vi "Liczniki.vi"() -> ()   [LabVIEW 2017, in "GUI.lvlib"]
uses:
  Libraries/GUI/GUI.lvlib
  <vilib>/Utility/config.llb/NI_LVConfig.lvlib
panel:
  out "Slave 2":T1
  out "Slave 6":T2
  out "Slave 4":T3
  out "Slave 3":T4
  out "Slave 5":T5
  in  "P_Sx":T6
  in  "stop":bool
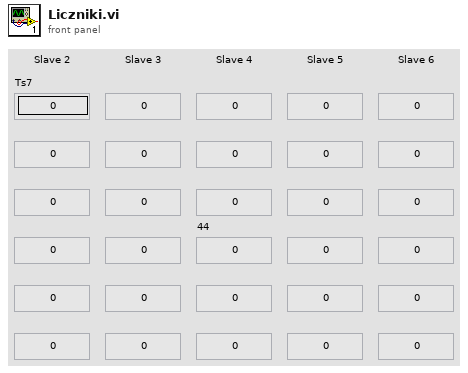
[diagram p1: front panel]
types:
  T1 = cluster{"Zmienna 11":dbl, "Zmienna 12":dbl, "Zmienna 13":dbl, "Zmienna 14":dbl, "Zmienna 15":dbl, "Zmienna 16":dbl}
  T2 = cluster{"Zmienna 51":dbl, "Zmienna 52":dbl, "Zmienna 53":dbl, "Zmienna 54":dbl, "Zmienna 55":dbl, "Zmienna 56":dbl}
  T3 = cluster{"Zmienna 31":dbl, "Zmienna 32":dbl, "Zmienna 33":dbl, "Zmienna 34":dbl, "Zmienna 35":dbl, "Zmienna 36":dbl}
  T4 = cluster{"Zmienna 21":dbl, "Zmienna 22":dbl, "Zmienna 23":dbl, "Zmienna 24":dbl, "Zmienna 25":dbl, "Zmienna 26":dbl}
  T5 = cluster{"Zmienna 41":dbl, "Zmienna 42":dbl, "Zmienna 43":dbl, "Zmienna 44":dbl, "Zmienna 45":dbl, "Zmienna 46":dbl}
  T6 = cluster{"Stan 1":dbl, "Stan 2":dbl, "Stan 3":dbl, "Stan 4":dbl, "Stan 5":dbl, "Stan 6":dbl}
  T7 = cluster{"Controls[]":refnum<vi>[], "Controls[]":refnum<vi>[], "Controls[]":refnum<vi>[], "Controls[]":refnum<vi>[], "Controls[]":refnum<vi>[], "Controls[]":refnum<vi>[]}
  T8 = typedef "NI_LVConfig.lvlib/Config Data RefNum.ctl" = refnum<k1>
  T9 = cluster{"[0]":cluster{"Stan 1":dbl, "Stan 2":dbl, "Stan 3":dbl, "Stan 4":dbl, "Stan 5":dbl, "Stan 6":dbl}, "[1]":cluster{"Stan 1":dbl, "Stan 2":dbl, "Stan 3":dbl, "Stan 4":dbl, "Stan 5":dbl, "Stan 6":dbl}, "[2]":cluster{"Stan 1":dbl, "Stan 2":dbl, "Stan 3":dbl, "Stan 4":dbl, "Stan 5":dbl, "Stan 6":dbl}, "[3]":cluster{"Stan 1":dbl, "Stan 2":dbl, "Stan 3":dbl, "Stan 4":dbl, "Stan 5":dbl, "Stan 6":dbl}, "[4]":cluster{"Stan 1":dbl, "Stan 2":dbl, "Stan 3":dbl, "Stan 4":dbl, "Stan 5":dbl, "Stan 6":dbl}}
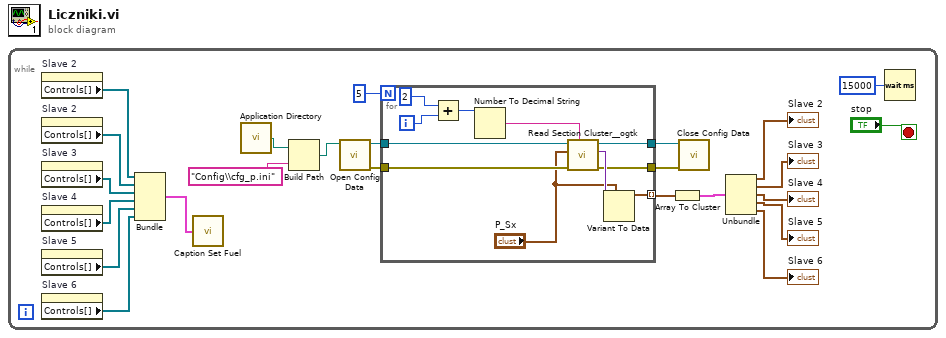
[diagram p0: block diagram]
diagram:
  n1 = while {
    stop <- "stop" stop-if-true
    n2 = property on="Slave 2" class="Clust (strict)"() -> ("Controls[]"=w1:refnum<vi>[])  [unwired: 2 in, 2 out]
    n3 = property on="Slave 2" class="Clust (strict)"() -> ("Controls[]"=w2:refnum<vi>[])  [unwired: 2 in, 2 out]
    n4 = property on="Slave 3" class="Clust (strict)"() -> ("Controls[]"=w3:refnum<vi>[])  [unwired: 2 in, 2 out]
    n5 = property on="Slave 4" class="Clust (strict)"() -> ("Controls[]"=w6:refnum<vi>[])  [unwired: 2 in, 2 out]
    n6 = property on="Slave 5" class="Clust (strict)"() -> ("Controls[]"=w5:refnum<vi>[])  [unwired: 2 in, 2 out]
    n7 = property on="Slave 6" class="Clust (strict)"() -> ("Controls[]"=w4:refnum<vi>[])  [unwired: 2 in, 2 out]
    n8 = Bundle("Controls[]"=w1, "Controls[]"=w2, "Controls[]"=w3, "Controls[]"=w6, "Controls[]"=w5, "Controls[]"=w4) -> (w7:T7)  [unwired: 1 in]
    n9 = call "Caption Set Fuel.vi"("Reference Cluster"=w7) -> ()
    n10 = call <vilib>:"Application Directory.vi"() -> ("Application Directory"=w22:path)
    n11 = Build Path(base path=w22, name or relative path="Config\\cfg_p.ini") -> (appended path=w20:path)
    n12 = call <vilib>:"Open Config Data.vi"("configuration file path"=w20) -> ("error out"=w18:errorcluster, "refnum"=w19:T8)  [unwired: 8 in, 1 out]
    n13 = for {
      N: 5 -> [_]
      tunnel: w19 -> [w34]
      tunnel: w18 -> [w33]
      tunnel: [w27] -> w16 mode=indexing
      tunnel: [w26] -> w9
      tunnel: [w25] -> w8
      i -> [w32]
      n14 = Add(x=2, y=w32) -> (x+y=w29:i32)
      n15 = Number To Decimal String(number=w29) -> (decimal integer string=w28:string)  [unwired: 1 in]
      n16 = call <userlib>:"Read Section Cluster__ogtk.vi"("section (optional)"=w28, "error in (no error)"=w33, "Section Formatted Cluster Type"="P_Sx", "refnum"=w34) -> ("error out"=w25:errorcluster, "Section Formatted Cluster"=w35:variant, "dup refnum"=w26:T8)  [unwired: 3 in, 2 out]
      n17 = Variant To Data(type="P_Sx", Variant=w35) -> (data=w27:T6)  [unwired: 1 in, 1 out]
    }
    n18 = Array To Cluster(array=w16) -> (cluster=w15:T9)
    n19 = call <vilib>:"Close Config Data.vi"("error in (no error)"=w8, "refnum"=w9) -> ()  [unwired: 8 in, 2 out]
    n20 = Unbundle(w15) -> ("[0]"=→"Slave 2":T6, "[1]"=→"Slave 3":T6, "[2]"=→"Slave 4":T6, "[3]"=→"Slave 5":T6, "[4]"=→"Slave 6":T6)
    n21 = Wait (ms)(milliseconds to wait=u32 15000) -> ()  [unwired: 1 out]
  }
